vi "校准记录写入.vi"(0 "MB session in":refnum<class "MB_Master.lvclass">, 1 "测量参数":u16(ring) items=["COD"=22, "氨氮"=3, "总氮"=2, "总磷"=1], 2 "测量模式":T1(ring), 3 "量程":enum16{"低量程", "高量程"}(ring), 5 "校准记录":T2, 11 "Error in":errorcluster caption="Error in (no error)") -> (4 "MB session out":refnum<class "MB_Master.lvclass">, 15 "error out":errorcluster)   [LabVIEW 2016, in "斯坦道CODcr.lvlib"]
uses:
  <vilib>/Plasmionique/MB Master/MB_Master/MB_Master.lvclass
  <vilib>/Plasmionique/MB Master/MB Master.lvlib
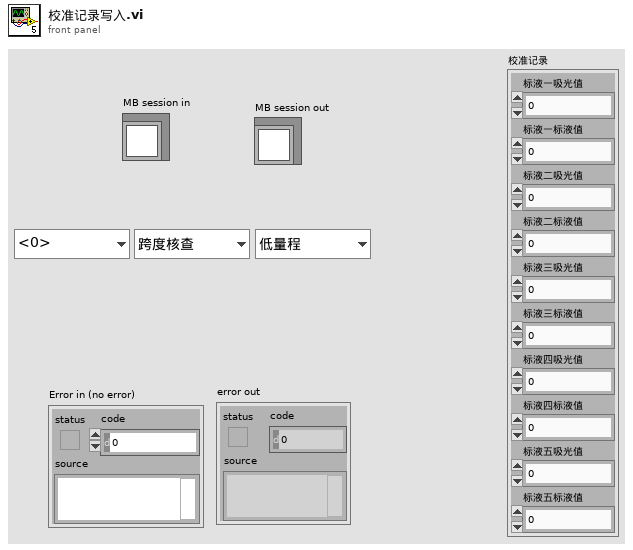
[diagram p1: front panel]
types:
  T1 = enum16{"跨度核查", "水样测量", "零点核查", "标样核查", "加标回收", "快捷测试", "空白校准", "标样校准"}
  T2 = cluster{"标液一吸光值":sgl, "标液一标液值":sgl, "标液二吸光值":sgl, "标液二标液值":sgl, "标液三吸光值":sgl, "标液三标液值":sgl, "标液四吸光值":sgl, "标液四标液值":sgl, "标液五吸光值":sgl, "标液五标液值":sgl}
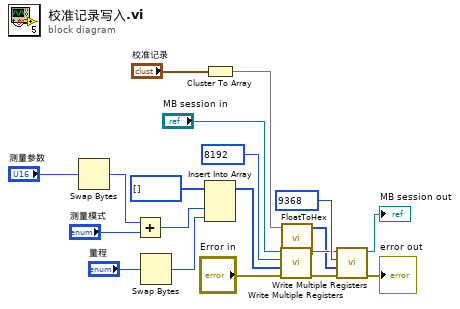
[diagram p0: block diagram]
diagram:
  n1 = Swap Bytes(anything="测量参数") -> (byte swapped=w14:u16)
  n2 = Add(x=w14, y="测量模式") -> (x+y=w16:u16)
  n3 = Swap Bytes(anything="量程") -> (byte swapped=w13:u16)
  n4 = Cluster To Array(cluster="校准记录") -> (array=w2:sgl[])
  n5 = Insert Into Array(array=u16[] [] ("数组"), new element #1=w16, new element #2=w13) -> (w9:u16[])  [unwired: 1 in]
  n6 = call <vilib>:"Write Multiple Registers.vi"("error in (no error)"="Error in", "values"=w9, "starting address"=u16 8192, "MB session in"="MB session in") -> ("error out"=w4:errorcluster, "MB session out"=w6:refnum<class "MB_Master.lvclass">)  [unwired: 6 in]
  n7 = call "FloatToHex.vi"("浮点数"=w2) -> ("DCBA整形输出"=w1:u16[])  [unwired: 10 in]
  n8 = call <vilib>:"Write Multiple Registers.vi"("error in (no error)"=w4, "values"=w1, "starting address"=u16 9368, "MB session in"=w6) -> ("error out"=→"error out":errorcluster, "MB session out"=→"MB session out":refnum<class "MB_Master.lvclass">)  [unwired: 6 in]
